vi "create book folder and path.vi"(5 "File Name":string="test", 7 "base path":path=path "C:/Users/gyue/Box/Guang Yue uiuc research box folder/data/Contour plot", 8 "error in":errorcluster, 11 "Book number":i32=545) -> (0 "error out":errorcluster, 1 "book name":string, 2 "appended path":path, 3 "timed File name":string)   [LabVIEW 2023]
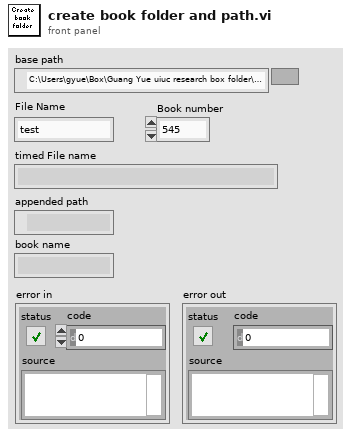
[diagram p1: front panel]
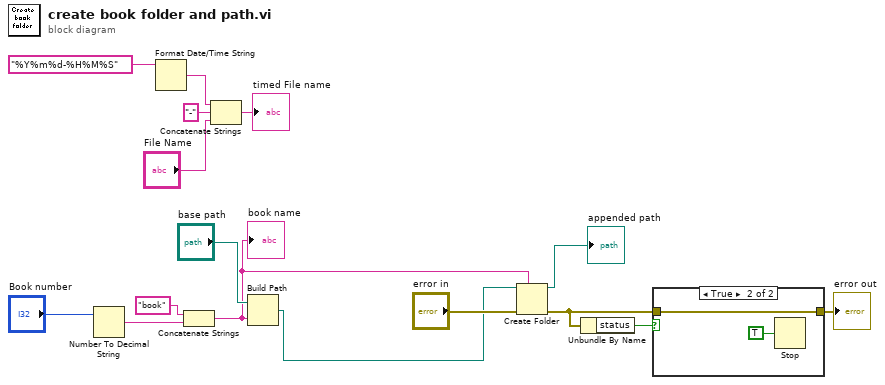
[diagram p0: block diagram]
diagram:
  n1 = Number To Decimal String(number="Book number") -> (decimal integer string=w11:string)  [unwired: 1 in]
  n2 = Format Date/Time String(time format string (%c)="%Y%m%d-%H%M%S") -> (date/time string=w16:string)  [unwired: 2 in]
  n3 = Concatenate Strings("book" ("string"), w11) -> (w3:string)
  "book name" <- w3
  n4 = Concatenate Strings(w16, "-" ("string"), "File Name") -> (→"timed File name":string)
  n5 = Build Path(base path="base path", name or relative path=w3) -> (appended path=w4:path)
  n6 = Create Folder(prompt (Create Folder)=w3, path (use dialog)=w4, error in="error in") -> (created path=→"appended path":path, error out=w6:errorcluster)  [unwired: 1 out]
  n7 = Unbundle By Name(w6) -> ("status"=w5:bool)
  n8 = case shown="True" w5 {
    tunnel: [w17 w19] -> w2
    tunnel: w6 -> [w17 w19]
    frame False {
    }
    frame True {
      n9 = Stop(stop? (T)=TRUE) -> ()
    }
  }
  "error out" <- w2
